vi "grab image (SubVI).vi"(8 "error in (no error)":errorcluster) -> (0 "error out":errorcluster, 3 "Refnum out":T1)   [LabVIEW 2013]
uses:
  <vilib>/vision/Image Controls.llb/IMAQ Image.ctl
  <vilib>/vision/driver/NI_Vision_Acquisition_Software.lvlib
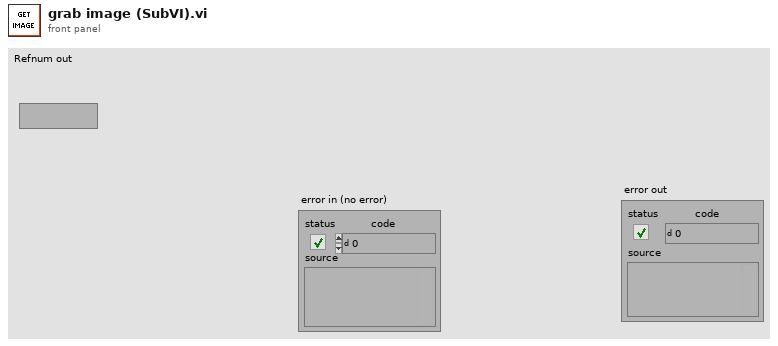
[diagram p1: front panel]
types:
  T1 = typedef "IMAQ Image.ctl" = refnum<image>
  T2 = typedef "Image Type" = u32
  T3 = typedef "IMAQdx.ctl" = refnum<k21>
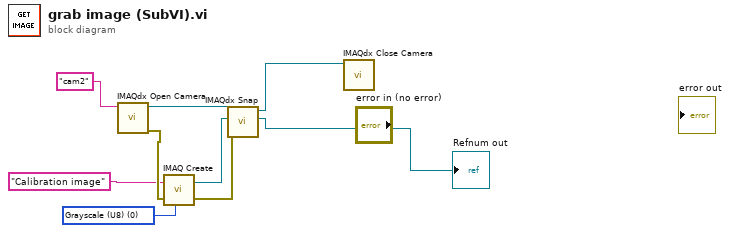
[diagram p0: block diagram]
diagram:
  w2 = T2 0 items=["Grayscale (U8)", "Grayscale (I16)", "Grayscale (SGL)", "Complex (CSG)", "RGB (U32)", "HSL (U32)", "RGB (U64)", "Grayscale (U16)"] ("Image Type")
  n1 = call <vilib>:"IMAQdx Open Camera.vi"("Session In"="cam2" ("Interface Name")) -> ("error out"=w8:errorcluster, "Session Out"=w7:T3)  [unwired: 9 in]
  n2 = call "IMAQ Create"("Image Name"="Calibration image", "Image Type"=w2, "error in (no error)"=w8) -> ("New Image"=w3:T1, "error out"=w4:errorcluster)  [unwired: 2 in]
  n3 = call <vilib>:"IMAQdx Snap.vi"("error in"=w4, "Image In"=w3, "Session In"=w7) -> ("Image Out"=→"Refnum out":T1, "Session Out"=w5:T3)  [unwired: 6 in, 1 out]
  n4 = call <vilib>:"IMAQdx Close Camera.vi"("Session In"=w5) -> ()  [unwired: 10 in, 1 out]
